vi "Update Terminal Size.vi"(8 "error in (no error)":errorcluster, 11 "Terminal in":refnum<class "Terminal.lvclass">) -> (0 "error out":errorcluster, 3 "Terminal out":refnum<class "Terminal.lvclass">)   [LabVIEW 2020, in "Terminal.lvlib" / "Terminal.lvclass"]
uses:
  Terminal.lvclass
  Terminal.lvclass/Terminal.ctl
  TermBuffer/TermBuffer.lvclass
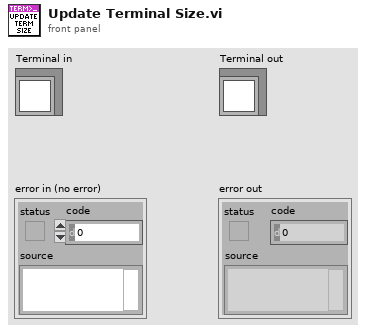
[diagram p1: front panel]
types:
  T1 = typedef "Terminal.lvlib/Terminal.lvclass/Ref Data.ctl" = cluster{"Connection":refnum<class "Connection.lvclass">, "Read Loop Running":bool, "Parse State":T2, "Terminal Options":T7, "Font Metrics":T10, "Scroll":i32}
  T2 = typedef "Terminal.lvlib/Terminal.lvclass/Parse State.ctl" = cluster{"Buffer State":T3, "Cursor":T4, "Attributes":T6}
  T3 = typedef "Terminal.lvlib/Terminal.lvclass/Buffer State.ctl" = cluster{"Sequence":string, "ESC":bool, "Alt Buf":bool}
  T4 = typedef "Terminal.lvlib/Terminal.lvclass/Cursor.ctl" = cluster{"Cur":T5, "Saved":T5}
  T5 = typedef "Terminal.lvlib/Terminal.lvclass/Position.ctl" = cluster{"Row":i32, "Col":i32}
  T6 = typedef "Terminal.lvlib/Text Attributes.ctl" = cluster{"FG":u32, "BG":u32, "Bold":bool, "Italic":bool, "Underline":bool, "Strike":bool, "Inverse":bool}
  T7 = typedef "Terminal.lvlib/Terminal Options.ctl" = cluster{"Implied CR with LF":bool, "Local Echo":bool, "Tab Width":i32, "Color Scheme":T8, "Default FG":T9, "Default BG":T9, "History Length":i32, "Font Face":string, "Font Size":i16, "Rows":i32, "Cols":i32}
  T8 = typedef "Terminal.lvlib/Color Scheme.ctl" = cluster{"Black":u32, "Red":u32, "Green":u32, "Yellow":u32, "Blue":u32, "Magenta":u32, "Cyan":u32, "White":u32, "Bright Black":u32, "Bright Red":u32, "Bright Green":u32, "Bright Yellow":u32, "Bright Blue":u32, "Bright Magenta":u32, "Bright Cyan":u32, "Bright White":u32}
  T9 = typedef "Terminal.lvlib/Color.ctl" = i8
  T10 = typedef "Terminal.lvlib/Terminal.lvclass/Font Metrics.ctl" = cluster{"Width":i16, "Height":i16}
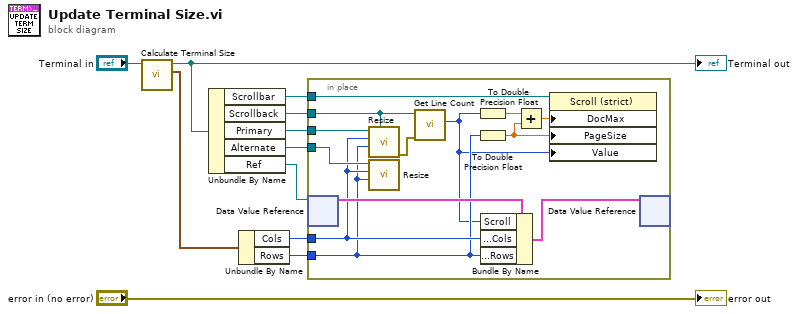
[diagram p0: block diagram]
diagram:
  n1 = call "Calculate Terminal Size.vi"("Terminal in"="Terminal in") -> ("Terminal Size"=w4:cluster{"Cols":u32, "Rows":u32}, "Terminal out"=w1:refnum<class "Terminal.lvclass">)  [unwired: 8 in, 1 out]
  "Terminal out" <- w1
  n2 = Unbundle By Name(w1) -> ("Scrollbar"=w2:refnum<vi>, "Scrollback"=w8:refnum<class "TermBuffer.lvclass">, "Primary"=w7:refnum<class "TermBuffer.lvclass">, "Alternate"=w6:refnum<class "TermBuffer.lvclass">, "Ref"=w3:refnum<data-value>)
  n3 = Unbundle By Name(w4) -> ("Cols"=w10:u32, "Rows"=w9:u32)
  n4 = in-place {
    in-place-border: w10 -> [w20]
    in-place-border: w9 -> [w13]
    in-place-border: w8 -> [w19]
    in-place-border: w7 -> [w22]
    in-place-border: w6 -> [w21]
    in-place-border: w2 -> [w14]
    n5 = in-place-dvr #1(w3) -> (w24:T1)  [unwired: 1 out]
    n6 = call "Resize.vi"("Scrollback"=w19, "Rows"=w13, "Cols"=w20, "TermBuffer in"=w22) -> ("error out"=w18:errorcluster)  [unwired: 6 in, 1 out]
    n7 = call "Resize.vi"("Rows"=w13, "Cols"=w20, "TermBuffer in"=w21) -> ()  [unwired: 7 in, 2 out]
    n8 = call "Get Line Count.vi"("error in (no error)"=w18, "TermBuffer in"=w19) -> ("Line Count"=w12:i32)  [unwired: 7 in, 2 out]
    n9 = To Double Precision Float(number=w12) -> (double precision float=w15:dbl)
    n10 = To Double Precision Float(number=w13) -> (double precision float=w16:dbl)
    n11 = Bundle By Name(cluster=w24, "Scroll"=w12, "Terminal Options.Cols"=w20, "Terminal Options.Rows"=w13) -> (w23:T1)
    n12 = Add(x=w15, y=w16) -> (x+y=w17:dbl)
    n13 = property class="Scroll (strict)"(reference=w14, "DocMax"=w17, "PageSize"=w16, "Value"=w12) -> ()  [unwired: 1 in, 2 out]
    n14 = in-place-dvr #1(w23) -> ()  [unwired: 2 out]
  }
  "error out" <- "error in (no error)"
